vi "Datacluster initialize.vi"(7 "show files in":cluster{"String":string, bool, i32, i32, dbl}[](array[cluster]), 9 "data names":string[](array[string]), 10 "data cluster":cluster{"all data":dbl[][]}[](array[cluster]), 11 "reset":bool) -> (3 "show files out":cluster{"String":string, bool, i32, i32, dbl}[](array[cluster]))   [LabVIEW 2019]
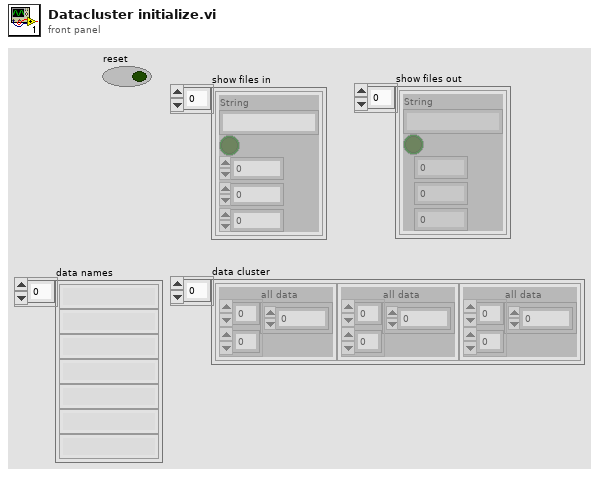
[diagram p1: front panel]
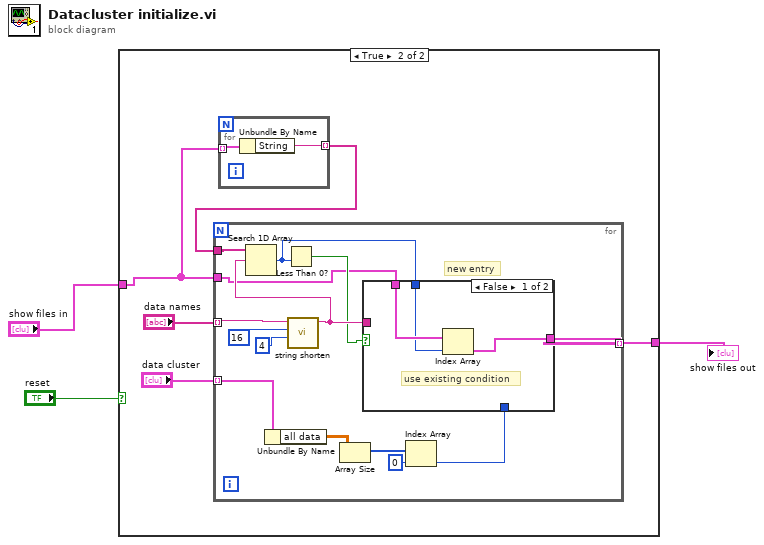
[diagram p0: block diagram]
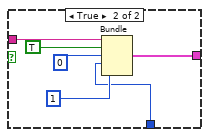
[diagram p3: hidden frame]
diagram:
  n1 = case shown="True" "reset" {
    tunnel: [w4 w7] -> w2
    tunnel: "show files in" -> [w4 w6]
    frame False {
    }
    frame True {
      n2 = for {
        tunnel: w6 -> [w11] mode=indexing
        tunnel: [w10] -> w5 mode=indexing
        n3 = Unbundle By Name(w11) -> ("String"=w10:string)
      }
      n4 = for {
        tunnel: [w25] -> w7 mode=indexing
        tunnel: "data names" -> [w17] mode=indexing
        tunnel: "data cluster" -> [w20] mode=indexing
        tunnel: w6 -> [w13]
        tunnel: w5 -> [w16]
        # "new entry"
        n5 = Unbundle By Name(w20) -> ("all data"=w24:dbl[][])
        n6 = call "string shorten.vi"("# of characters in the beginning"=4, "# of characters in the end"=16, "input"=w17) -> ("shortened"=w15:string)  [unwired: 8 in]
        n7 = Search 1D Array(1D array=w16, element=w15) -> (index of element=w12:i32)  [unwired: 1 in]
        n8 = Less Than 0?(x=w12) -> (x < 0?=w14:bool)
        n9 = Array Size(array=w24) -> (size(s)=w23:i32[])
        n10 = Index Array(array=w23, index=0) -> (element=w21:i32)
        n11 = case shown="False" w14 {
          tunnel: [w26 w34] -> w25
          tunnel: w21 -> [_ w31]
          tunnel: w15 -> [_ w30]
          tunnel: w13 -> [w28 _]
          tunnel: w12 -> [w27 _]
          frame False {
            # "use existing condition"
            n12 = Index Array(array=w28, index=w27) -> (element=w26:cluster{"String":string, bool, i32, i32, dbl})
          }
          frame True {
            n13 = Bundle("shortened"=w30, TRUE, 0, w31, 1) -> (w34:cluster{"shortened":string, bool, i32, i32, i32})  [unwired: 1 out]
          }
        }
      }
    }
  }
  "show files out" <- w2
